vi "sum( I exp( i holo ) ).vi"(9 "Spot(n-1) holo":cdb[](array[numeric]), 10 "Spot(n) Intensity":dbl, 11 "Spot(n) Holo":u8[](array[numeric])) -> (3 "holo_mod":cdb[](array[numeric]))   [LabVIEW 2020]
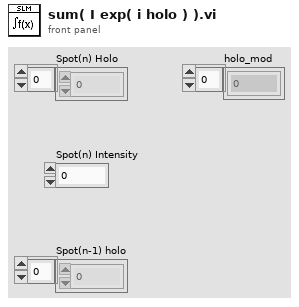
[diagram p1: front panel]
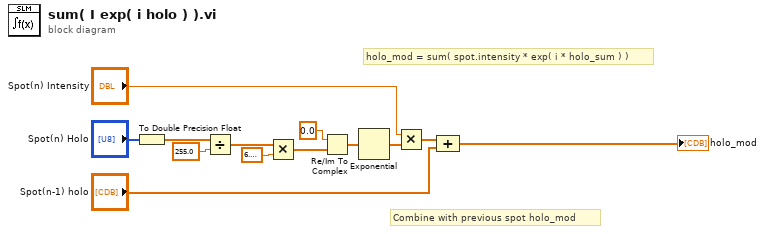
[diagram p0: block diagram]
diagram:
  # "Combine with previous spot holo_mod"
  # "holo_mod = sum( spot.intensity * exp( i * holo_sum ) )"
  n1 = To Double Precision Float(number="Spot(n) Holo") -> (double precision float=w13:dbl[])
  n2 = Divide(x=w13, y=255.0) -> (x/y=w3:dbl[])
  n3 = Multiply(x=w3, y=6.283185307179586) -> (x*y=w7:dbl[])
  n4 = Re/Im To Complex(1:w7, 2:0.0 ("x")) -> (0:w2:cdb[])
  n5 = Exponential(1:w2) -> (0:w8:cdb[])
  n6 = Multiply(x="Spot(n) Intensity", y=w8) -> (x*y=w9:cdb[])
  n7 = Compound Arithmetic op=ADD(w9, "Spot(n-1) holo") -> (→"holo_mod":cdb[])
